vi "Test Solenoids.vi"(10 "Input":bool=TRUE, 11 "Solenoid":i32) -> ()   [LabVIEW 2014]
uses:
  <vilib>/Rock Robotics/WPI/Solenoid/WPI_SolenoidValue.ctl
  <vilib>/Rock Robotics/WPI/Solenoid/WPI_SolenoidSetEnum.vi
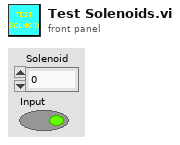
[diagram p1: front panel]
types:
  T1 = typedef "WPI_SolenoidValue.ctl" = enum16{"Off", "On", "Forward", "Reverse"}
  T2 = typedef "WPI_SolenoidDevRef.ctl" = cluster{"DevStatus":errorcluster, "Pneumatics Control Module":u8, "Forward Solenoid Channel":T3, "Reverse Solenoid Channel":T3}
  T3 = typedef "WPI_SolenoidChannel.ctl" = enum8{"Solenoid 0", "Solenoid 1", "Solenoid 2", "Solenoid 3", "Solenoid 4", "Solenoid 5", "Solenoid 6", "Solenoid 7", "Invalid"}
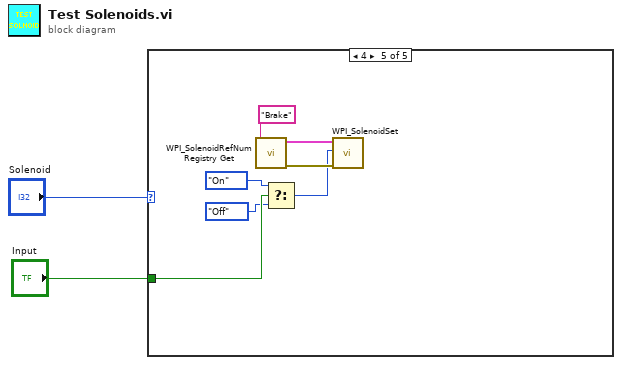
[diagram p0: block diagram]
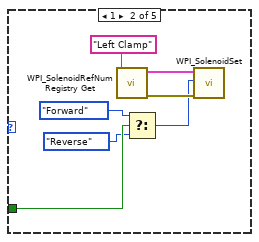
[diagram p3: hidden frame]
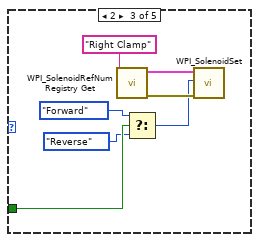
[diagram p4: hidden frame]
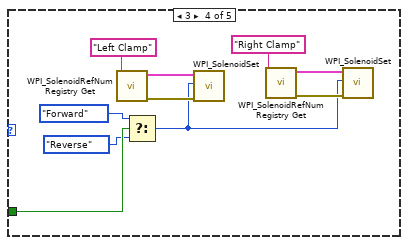
[diagram p5: hidden frame]
diagram:
  n1 = case shown="4" "Solenoid" {
    tunnel: "Input" -> [_ w5 w12 w23 w30]
    frame 0, Default {
    }
    frame 1 {
      n2 = call <vilib>:"WPI_SolenoidRefNum Registry Get.vi"("refnum name"="Left Clamp") -> ("error out"=w8:errorcluster, "SolenoidDevRef"=w7:T2)  [unwired: 9 in]
      n3 = Select(t=WPI_SolenoidValue."Forward" ("Value"), s=w5, f=WPI_SolenoidValue."Reverse" ("Value")) -> (s? t:f=w6:T1)
      n4 = call-poly <vilib>:"WPI_SolenoidSet.vi"("error in (no error)"=w8, "Value"=w6, "SolenoidDevRef"=w7) -> ()  [unwired: 7 in, 2 out]
    }
    frame 2 {
      n5 = call <vilib>:"WPI_SolenoidRefNum Registry Get.vi"("refnum name"="Right Clamp") -> ("error out"=w15:errorcluster, "SolenoidDevRef"=w14:T2)  [unwired: 9 in]
      n6 = Select(t=WPI_SolenoidValue."Forward" ("Value"), s=w12, f=WPI_SolenoidValue."Reverse" ("Value")) -> (s? t:f=w13:T1)
      n7 = call-poly <vilib>:"WPI_SolenoidSet.vi"("error in (no error)"=w15, "Value"=w13, "SolenoidDevRef"=w14) -> ()  [unwired: 7 in, 2 out]
    }
    frame 3 {
      n8 = call <vilib>:"WPI_SolenoidRefNum Registry Get.vi"("refnum name"="Left Clamp") -> ("error out"=w25:errorcluster, "SolenoidDevRef"=w24:T2)  [unwired: 9 in]
      n9 = Select(t=WPI_SolenoidValue."Forward" ("Value"), s=w23, f=WPI_SolenoidValue."Reverse" ("Value")) -> (s? t:f=w17:T1)
      n10 = call-poly <vilib>:"WPI_SolenoidSet.vi"("error in (no error)"=w25, "Value"=w17, "SolenoidDevRef"=w24) -> ()  [unwired: 7 in, 2 out]
      n11 = call <vilib>:"WPI_SolenoidRefNum Registry Get.vi"("refnum name"="Right Clamp") -> ("error out"=w19:errorcluster, "SolenoidDevRef"=w20:T2)  [unwired: 9 in]
      n12 = call-poly <vilib>:"WPI_SolenoidSet.vi"("error in (no error)"=w19, "Value"=w17, "SolenoidDevRef"=w20) -> ()  [unwired: 7 in, 2 out]
    }
    frame 4 {
      n13 = call <vilib>:"WPI_SolenoidRefNum Registry Get.vi"("refnum name"="Brake") -> ("error out"=w32:errorcluster, "SolenoidDevRef"=w31:T2)  [unwired: 9 in]
      n14 = Select(t=WPI_SolenoidValue."On" ("Value"), s=w30, f=WPI_SolenoidValue."Off" ("Value")) -> (s? t:f=w27:T1)
      n15 = call-poly <vilib>:"WPI_SolenoidSet.vi"("error in (no error)"=w32, "Value"=w27, "SolenoidDevRef"=w31) -> ()  [unwired: 7 in, 2 out]
    }
  }
